vi "Angle Between 2D Vectors.vi"(10 "Array":dbl[](array[numeric]), 11 "Array 2":dbl[](array[numeric])) -> (3 "Numeric":dbl)   [LabVIEW 2023]
uses:
  <vilib>/Analysis/baseanly.llb/Real Dot Product.vi
  <vilib>/Analysis/NI_AALBase.lvlib
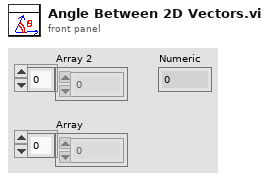
[diagram p1: front panel]
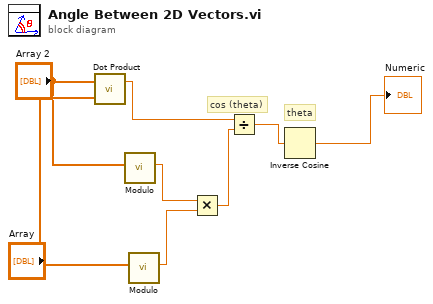
[diagram p0: block diagram]
diagram:
  # "theta"
  # "cos (theta)"
  n1 = call-poly <vilib>:"Dot Product.vi"("Y Vector"="Array", "X Vector"="Array 2") -> ("X * Y"=w5:dbl)  [unwired: 1 out]
  n2 = call "Modulo.vi"("2D vector"="Array 2") -> ("Modulo"=w3:dbl)  [unwired: 10 in]
  n3 = call "Modulo.vi"("2D vector"="Array") -> ("Modulo"=w4:dbl)  [unwired: 10 in]
  n4 = Multiply(x=w3, y=w4) -> (x*y=w6:dbl)
  n5 = Divide(x=w5, y=w6) -> (x/y=w7:dbl)
  n6 = Inverse Cosine(1:w7) -> (0:→"Numeric":dbl)
